vi "InverseKinematics_4Omni.vi"(0 "Vx":dbl, 1 "Robot Radius \n(0.157 m)":dbl=0.157, 2 "Wheel Radius\n(0.05 m)":dbl=0.05, 5 "Vy":dbl, 7 "Omega":dbl, 11 "error in (no error)":errorcluster) -> (4 "w1-FL":dbl, 6 "w2-BL":dbl, 8 "w3-FR":dbl, 10 "w4-BR":dbl, 15 "error out":errorcluster)   [LabVIEW 2017]
doc: "This VI create for 4 Omni-Wheel Robot that using to substract entire movement of robot (Vx, Vy, Omega) into movement of each motor (w1, w2, w3, w4) by InverseKinematics Formula \n\n----------------\nLast Modified on 18-04-2025 by kidsadoi"
panel:
  # "Input Position"
  # "Position Base on my Stupid Crab's Wheel"
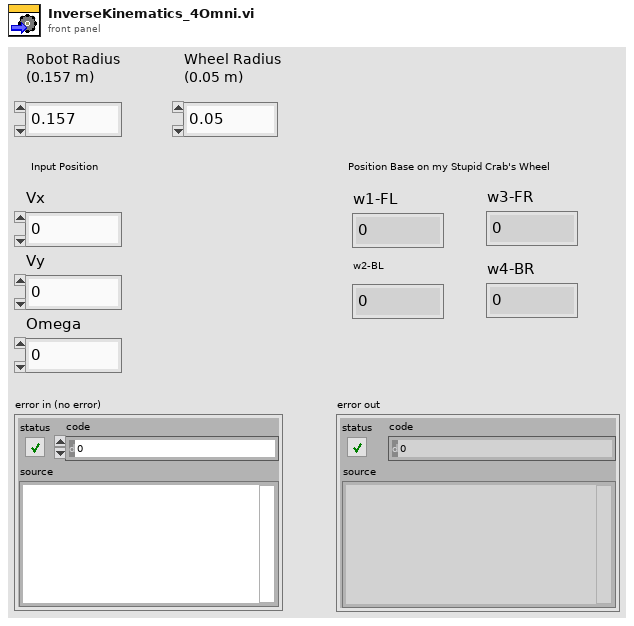
[diagram p1: front panel]
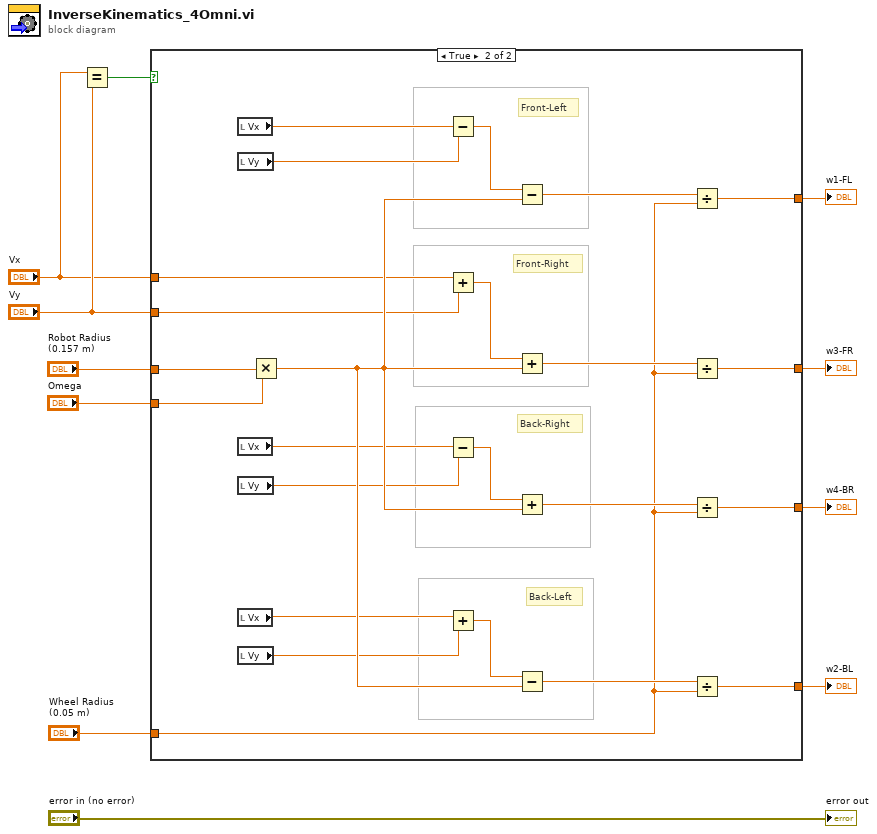
[diagram p0: block diagram]
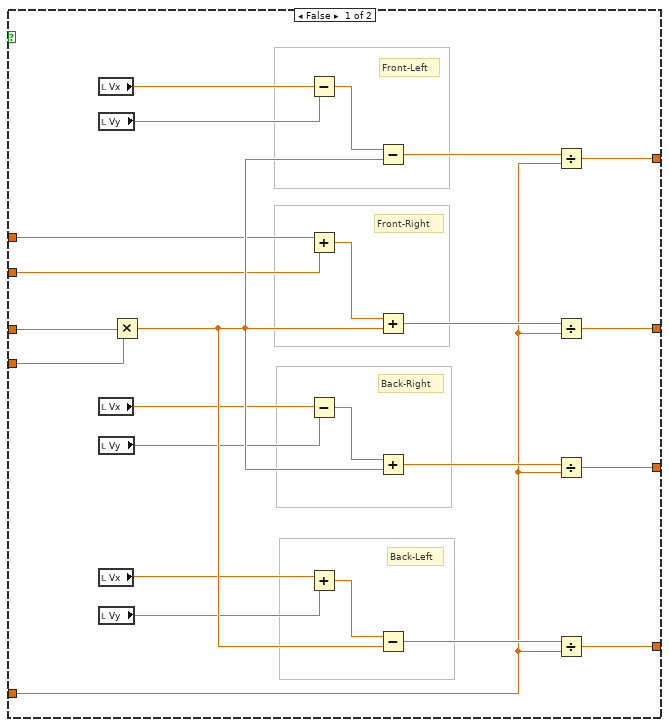
[diagram p2: hidden frame]
diagram:
  n1 = Equal?(x="Vx", y="Vy") -> (x = y?=w3:bool)
  n2 = case shown="True" w3 {
    tunnel: "Vy" -> [w20 w42]
    tunnel: "Vx" -> [w19 w41]
    tunnel: "Omega" -> [w18 w44]
    tunnel: "Robot Radius \n(0.157 m)" -> [w17 w43]
    tunnel: "Wheel Radius\n(0.05 m)" -> [w16 w40]
    tunnel: [w15 w36] -> w7
    tunnel: [w14 w37] -> w6
    tunnel: [w13 w38] -> w5
    tunnel: [w12 w39] -> w4
    frame False {
      # "Back-Left"
      # "Back-Right"
      # "Front-Right"
      # "Front-Left"
      n3 = local read "Vx"() -> (w22:dbl)
      n4 = local read "Vy"() -> (w21:dbl)
      n5 = local read "Vx"() -> (w23:dbl)
      n6 = local read "Vy"() -> (w24:dbl)
      n7 = local read "Vx"() -> (w25:dbl)
      n8 = local read "Vy"() -> (w26:dbl)
      n9 = Multiply(x=w17, y=w18) -> (x*y=w31:dbl)
      n10 = Subtract(x=w22, y=w21) -> (x-y=w34:dbl)
      n11 = Add(x=w19, y=w20) -> (x+y=w35:dbl)
      n12 = Subtract(x=w23, y=w24) -> (x-y=w32:dbl)
      n13 = Add(x=w25, y=w26) -> (x+y=w33:dbl)
      n14 = Subtract(x=w34, y=w31) -> (x-y=w27:dbl)
      n15 = Add(x=w35, y=w31) -> (x+y=w28:dbl)
      n16 = Add(x=w32, y=w31) -> (x+y=w29:dbl)
      n17 = Subtract(x=w33, y=w31) -> (x-y=w30:dbl)
      n18 = Divide(x=w27, y=w16) -> (x/y=w12:dbl)
      n19 = Divide(x=w28, y=w16) -> (x/y=w13:dbl)
      n20 = Divide(x=w29, y=w16) -> (x/y=w14:dbl)
      n21 = Divide(x=w30, y=w16) -> (x/y=w15:dbl)
    }
    frame True {
      # "Back-Left"
      # "Back-Right"
      # "Front-Right"
      # "Front-Left"
      n22 = local read "Vx"() -> (w46:dbl)
      n23 = local read "Vy"() -> (w45:dbl)
      n24 = local read "Vx"() -> (w47:dbl)
      n25 = local read "Vy"() -> (w48:dbl)
      n26 = local read "Vx"() -> (w49:dbl)
      n27 = local read "Vy"() -> (w50:dbl)
      n28 = Multiply(x=w43, y=w44) -> (x*y=w55:dbl)
      n29 = Subtract(x=w46, y=w45) -> (x-y=w58:dbl)
      n30 = Add(x=w41, y=w42) -> (x+y=w59:dbl)
      n31 = Subtract(x=w47, y=w48) -> (x-y=w56:dbl)
      n32 = Add(x=w49, y=w50) -> (x+y=w57:dbl)
      n33 = Subtract(x=w58, y=w55) -> (x-y=w51:dbl)
      n34 = Add(x=w59, y=w55) -> (x+y=w52:dbl)
      n35 = Add(x=w56, y=w55) -> (x+y=w53:dbl)
      n36 = Subtract(x=w57, y=w55) -> (x-y=w54:dbl)
      n37 = Divide(x=w51, y=w40) -> (x/y=w39:dbl)
      n38 = Divide(x=w52, y=w40) -> (x/y=w38:dbl)
      n39 = Divide(x=w53, y=w40) -> (x/y=w37:dbl)
      n40 = Divide(x=w54, y=w40) -> (x/y=w36:dbl)
    }
  }
  "w1-FL" <- w4
  "w3-FR" <- w5
  "w4-BR" <- w6
  "w2-BL" <- w7
  "error out" <- "error in (no error)"
